vi "main.vi"() -> ()   [LabVIEW 2026]
uses:
  Dependencies/data.ctl
  Dependencies/dependencies.lvlib
panel:
  out "Cluster":T1
  in  "Numeric":dbl
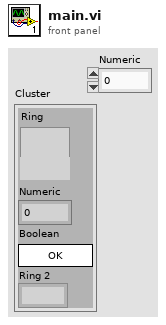
[diagram p1: front panel]
types:
  T1 = typedef "dependencies.lvlib/data.ctl" = cluster{"Ring":u16, "Numeric":dbl, "Boolean":bool, "Ring 2":u16}
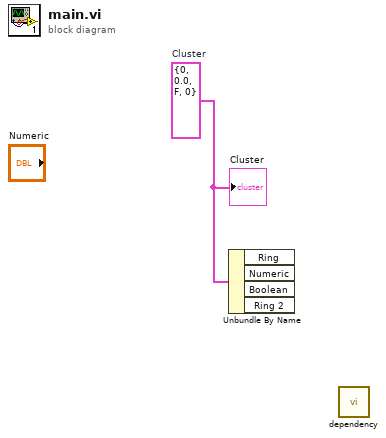
[diagram p0: block diagram]
diagram:
  w1 = T1 {"Ring"=0, "Numeric"=0.0, "Boolean"=FALSE, "Ring 2"=0}  # Cluster
  n1 = Unbundle By Name(w1) -> ()  [unwired: 4 out]
  n2 = call "dependency.vi"() -> ()  [unwired: 11 in, 1 out]
  "Cluster" <- w1
